vi "USB-4000 MultiAi - ExtTrig.vi"() -> ()   [LabVIEW 2016]
panel:
  in  "TrigEdge":u8(ring)=1 items=["下降沿", "上升沿"]
  out "数值":i32
  in  "Range":sgl=10.0
  out "error out":errorcluster caption="错误输出"
  in  "停止":bool
  out "波形图":cluster{dbl, dbl, sgl[][]}(graph)
  in  "读取通道选择":T1={"CH 0"=TRUE, "CH 1"=TRUE, "CH 2"=TRUE, "CH 3"=TRUE, "CH 4"=TRUE, "CH 5"=TRUE, "CH 6"=TRUE, "CH 7"=TRUE, "CH 8"=FALSE, "CH 9"=FALSE, "CH 10"=FALSE, "CH 11"=FALSE, "CH 12"=FALSE, "CH 13"=FALSE, "CH 14"=FALSE, "CH 15"=FALSE}
  in  "Num":u32=50000 caption="每通道读取点数"
  in  "SampleRate":u32=500000 caption="SampleRate (pts/s)"
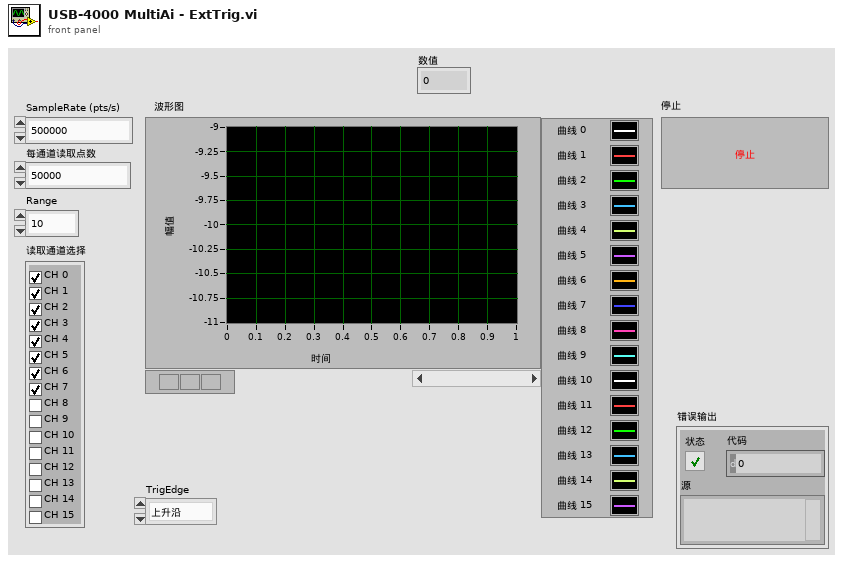
[diagram p1: front panel]
types:
  T1 = cluster{"CH 0":bool, "CH 1":bool, "CH 2":bool, "CH 3":bool, "CH 4":bool, "CH 5":bool, "CH 6":bool, "CH 7":bool, "CH 8":bool, "CH 9":bool, "CH 10":bool, "CH 11":bool, "CH 12":bool, "CH 13":bool, "CH 14":bool, "CH 15":bool}
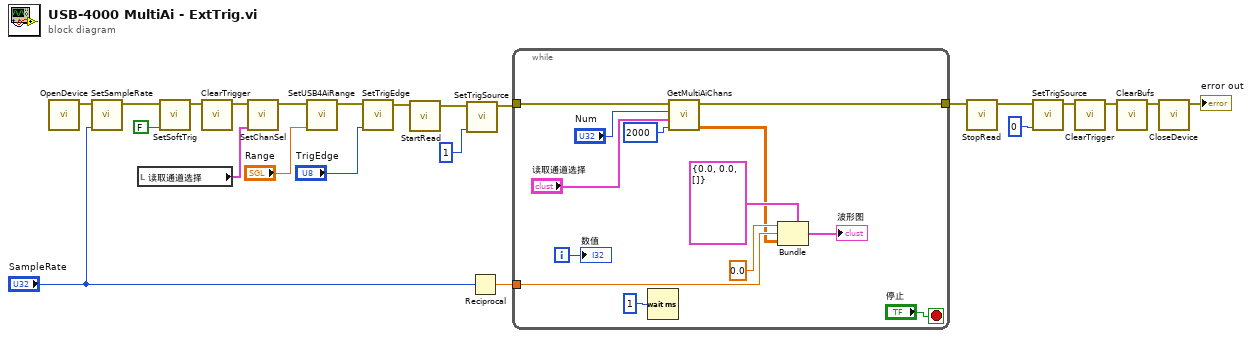
[diagram p0: block diagram]
diagram:
  n1 = call "OpenDevice.vi"() -> ("error out"=w23:errorcluster)  [unwired: 11 in]
  n2 = call "SetSampleRate.vi"("SampleRate"="SampleRate", "error in"=w23) -> ("error out"=w14:errorcluster)  [unwired: 9 in]
  n3 = local read "读取通道选择"() -> (w18:T1)
  n4 = call "SetSoftTrig.vi"("SoftTrig"=FALSE, "error in"=w14) -> ("error out"=w9:errorcluster)  [unwired: 9 in]
  n5 = call "ClearTrigger.vi"("错误输入（无错误）"=w9) -> ("错误输出"=w8:errorcluster)  [unwired: 10 in]
  n6 = call "SetChanSel.vi"("读取通道选择"=w18, "错误输入"=w8) -> ("错误输出"=w19:errorcluster)  [unwired: 9 in]
  n7 = call "SetUSB4AiRange.vi"("Range"="Range", "error in"=w19) -> ("error out"=w7:errorcluster)  [unwired: 9 in]
  n8 = call "SetTrigEdge.vi"("TrigEdge"="TrigEdge", "错误输入（无错误）"=w7) -> ("错误输出"=w3:errorcluster)  [unwired: 9 in]
  n9 = call "StartRead.vi"("error in"=w3) -> ("error out"=w2:errorcluster)  [unwired: 10 in]
  n10 = call "SetTrigSource.vi"("TrigSource"=u8 1, "error in"=w2) -> ("error out"=w1:errorcluster)  [unwired: 9 in]
  n11 = Reciprocal(x="SampleRate") -> (1/x=w13:dbl)
  n12 = while {
    tunnel: w13 -> [w35]
    tunnel: w1 -> [w36]
    tunnel: [w34] -> w12
    i -> [w25]
    stop <- "停止" stop-if-true
    n13 = Wait (ms)(milliseconds to wait=u32 1 ("等待时间（毫秒）")) -> ()  [unwired: 1 out]
    n14 = call "GetMultiAiChans.vi"("TimeOut (ms)"=2000, "ChansSel"="读取通道选择", "Num"="Num", "error in"=w36) -> ("Data"=w26:sgl[][], "error out"=w34:errorcluster)  [unwired: 6 in]
    n15 = Bundle(cluster=cluster{dbl, dbl, sgl[][]} {0.0, 0.0, []}, 0.0, w35, w26) -> (→"波形图":cluster{dbl, dbl, sgl[][]})
    "数值" <- w25
  }
  n16 = call "StopRead.vi"("error in"=w12) -> ("error out"=w10:errorcluster)  [unwired: 10 in]
  n17 = call "SetTrigSource.vi"("TrigSource"=u8 0, "error in"=w10) -> ("error out"=w5:errorcluster)  [unwired: 9 in]
  n18 = call "ClearTrigger.vi"("错误输入（无错误）"=w5) -> ("错误输出"=w4:errorcluster)  [unwired: 10 in]
  n19 = call "ClearBufs.vi"("error in"=w4) -> ("error out"=w22:errorcluster)  [unwired: 10 in]
  n20 = call "CloseDevice.vi"("error in"=w22) -> ("error out"=→"error out":errorcluster)  [unwired: 10 in]
